vi "Write to File.vi"(7 "Section Name":string, 8 "error in (no error)":errorcluster, 10 "INI Ref":T1, 11 "Numeric Assertion in":refnum<class "Numeric Assertion.lvclass">) -> (0 "error out":errorcluster, 2 "INI Ref out":T1, 3 "Numeric Assertion out":refnum<class "Numeric Assertion.lvclass">)   [LabVIEW 2020, in "MacroAssert.lvlib" / "Numeric Assertion.lvclass"]
doc: "Writes associated parameters to the file identified by <B>INI Ref</B>."
uses:
  Numeric Assertion.lvclass
  <vilib>/Utility/config.llb/Config Data RefNum.ctl
  <vilib>/Utility/error.llb/Error Cluster From Error Code.vi
  <vilib>/Utility/config.llb/Write Key (String).vi
  <vilib>/Utility/config.llb/Write Key (Double).vi
  Assertion Step/Assertion Step.lvclass
  SubVIs/Custom Errors/Custom Errors.lvlib
  <vilib>/Utility/config.llb/NI_LVConfig.lvlib
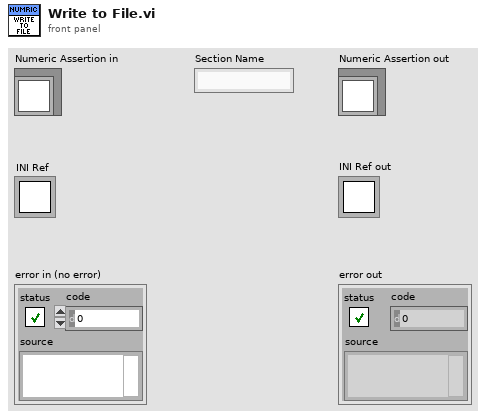
[diagram p1: front panel]
types:
  T1 = typedef "NI_LVConfig.lvlib/Config Data RefNum.ctl" = refnum<k1>
  T2 = typedef "MacroAssert.lvlib/Numeric Assertion.lvclass/Numeric Assertion Type.ctl" = enum16{"Numeric Ctl Value", "Array Ctl Size", "Ctl Width Property", "Ctl Height Property", "VI Width", "VI Height", "Window Width", "Window Height", "Window Scale", "Number of Monitors"}
  T3 = typedef "MacroAssert.lvlib/Numeric Assertion.lvclass/Numeric Comparator.ctl" = enum16{"Equals", "Is greater than", "Is greater than or equal to", "Is less than", "Is less than or equal to", "Does not equal"}
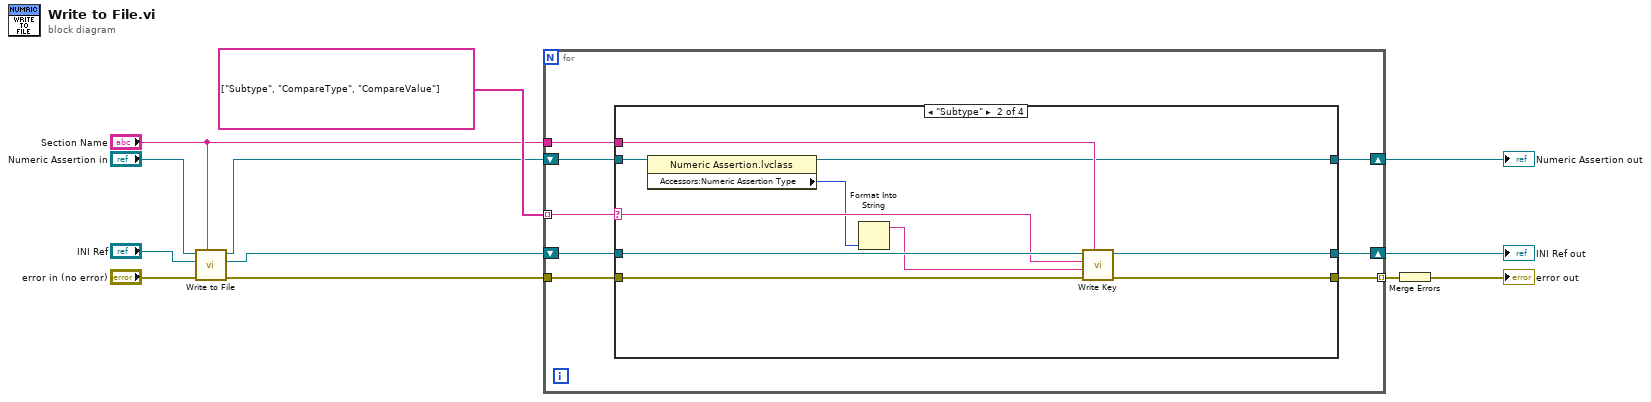
[diagram p0: block diagram]
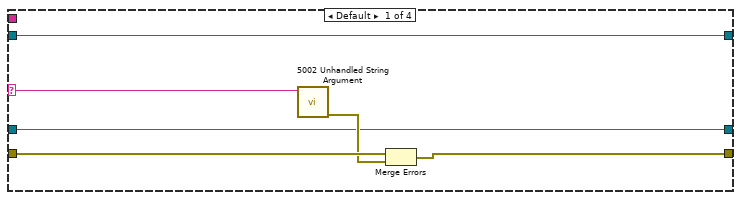
[diagram p2: hidden frame]
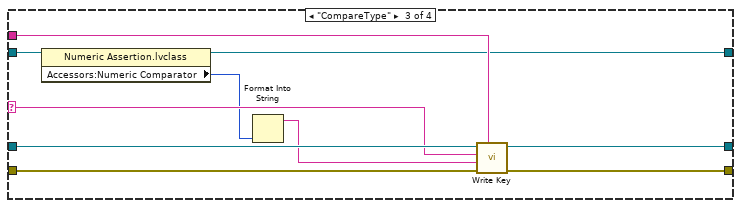
[diagram p3: hidden frame]
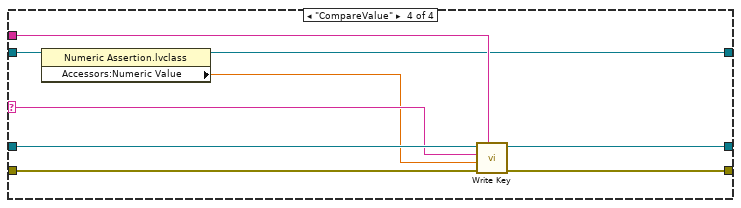
[diagram p4: hidden frame]
diagram:
  n1 = call-parent "Write to File.vi"("Section Name"="Section Name", "error in (no error)"="error in (no error)", "INI Ref"="INI Ref", "Assertion Step in"="Numeric Assertion in") -> ("error out"=w12:errorcluster, "INI Ref out"=w9:T1, "Assertion Step out"=w4:refnum<class "Numeric Assertion.lvclass">)  [unwired: 5 in]
  n2 = for {
    tunnel: string[] ["Subtype", "CompareType", "CompareValue"] -> [w16] mode=indexing
    tunnel: w12 -> [w20]
    tunnel: "Section Name" -> [w15]
    shift-right: [w13] -> w2
    shift-left: w4 -> [w14]
    tunnel: [w19] -> w5 mode=indexing
    shift-right: [w17] -> w8
    shift-left: w9 -> [w18]
    n3 = case shown="\"Subtype\"" w16 {
      selector: w16 -> [w21 w31 w41 w50]
      tunnel: w20 -> [w26 w36 w46 w55]
      tunnel: w15 -> [_ w32 w42 w51]
      tunnel: w14 -> [w22 w30 w40 w49]
      tunnel: [w22 w27 w37 w48] -> w13
      tunnel: [w24 w35 w45 w54] -> w19
      tunnel: w18 -> [w23 w34 w44 w53]
      tunnel: [w23 w33 w43 w52] -> w17
      frame Default {
        n4 = call "5002 Unhandled String Argument.vi"("Argument"=w21) -> ("error out"=w25:errorcluster)  [unwired: 10 in]
        n5 = Merge Errors(w26, w25) -> (w24:errorcluster)
      }
      frame "Subtype" {
        n6 = property class="Numeric Assertion.lvclass"(reference=w30) -> (reference out=w27:refnum<class "Numeric Assertion.lvclass">, "Accessors:Numeric Assertion Type"=w29:T2)  [unwired: 1 in, 1 out]
        n7 = Format Into String(w29) -> (resulting string=w28:string)  [unwired: 3 in, 1 out]
        n8 = call-poly <vilib>:"Write Key.vi"("section"=w32, "error in (no error)"=w36, "value"=w28, "key"=w31, "refnum"=w34) -> ("error out"=w35:errorcluster, "refnum out"=w33:T1)  [unwired: 4 in, 1 out]
      }
      frame "CompareType" {
        n9 = property class="Numeric Assertion.lvclass"(reference=w40) -> (reference out=w37:refnum<class "Numeric Assertion.lvclass">, "Accessors:Numeric Comparator"=w39:T3)  [unwired: 1 in, 1 out]
        n10 = Format Into String(w39) -> (resulting string=w38:string)  [unwired: 3 in, 1 out]
        n11 = call-poly <vilib>:"Write Key.vi"("section"=w42, "error in (no error)"=w46, "value"=w38, "key"=w41, "refnum"=w44) -> ("error out"=w45:errorcluster, "refnum out"=w43:T1)  [unwired: 4 in, 1 out]
      }
      frame "CompareValue" {
        n12 = property class="Numeric Assertion.lvclass"(reference=w49) -> (reference out=w48:refnum<class "Numeric Assertion.lvclass">, "Accessors:Numeric Value"=w47:dbl)  [unwired: 1 in, 1 out]
        n13 = call-poly <vilib>:"Write Key.vi"("section"=w51, "error in (no error)"=w55, "value"=w47, "key"=w50, "refnum"=w53) -> ("error out"=w54:errorcluster, "refnum out"=w52:T1)  [unwired: 4 in, 1 out]
      }
    }
  }
  "Numeric Assertion out" <- w2
  "INI Ref out" <- w8
  n14 = Merge Errors(w5) -> (→"error out":errorcluster)
